vi "Retrive Data.vi"(8 "error in (no error)":errorcluster, 9 "Tag":string, 10 "Tree In":refnum<class "Tree.lvclass">, 11 "Tree Data in":refnum<class "Tree Data.lvclass">) -> (0 "error out":errorcluster, 1 "Data Out":T1, 2 "Tree Out":refnum<class "Tree.lvclass">, 3 "Tree Data out":refnum<class "Tree Data.lvclass">, 5 "Data Group Out":T1[](array[typedef]))   [LabVIEW 2024, in "Tree Data.lvclass"]
uses:
  Tree Data.lvclass
  Tree/Tree.lvclass
  Tree/Type Def/Tree Item.ctl
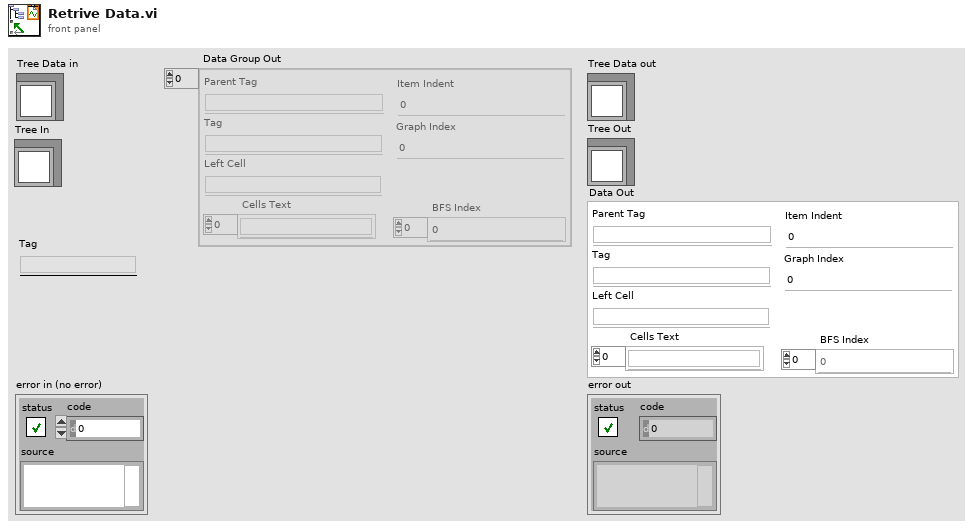
[diagram p1: front panel]
types:
  T1 = typedef "Tree Item.ctl" = cluster{"Parent Tag":string, "Tag":string, "Left Cell":string, "Cells Text":string[], "BFS Index":i32[], "Graph Index":i32, "Item Indent":i32}
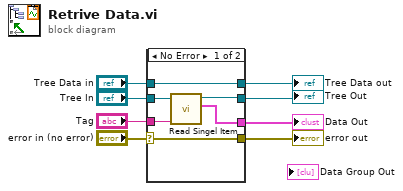
[diagram p0: block diagram]
diagram:
  n1 = case shown="No Error" "error in (no error)" {
    selector: "error in (no error)" -> [w13 w17]
    tunnel: [w13 w17] -> w7
    tunnel: [w14 w16] -> w5
    tunnel: "Tree Data in" -> [w14 w16]
    tunnel: "Tree In" -> [w12 w15]
    tunnel: [w10 w15] -> w3
    tunnel: "Tag" -> [w11 _]
    tunnel: [w9 _] -> w1
    frame No Error {
      n2 = call "Read Singel Item.vi"("Tag"=w11, "Tree in"=w12) -> ("Element Out"=w9:T1, "Tree out"=w10:refnum<class "Tree.lvclass">)  [unwired: 8 in]
    }
    frame Error {
    }
  }
  "error out" <- w7
  "Tree Data out" <- w5
  "Tree Out" <- w3
  "Data Out" <- w1
